vi "Live_Update_Bollean_indicator.vi"(8 "error in (no error)":errorcluster, 10 "Array 2":bool[](array[boolean]), 11 "Array":refnum<vi>[](array[refnum])) -> ()   [LabVIEW 2017]
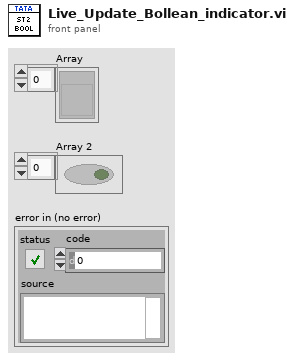
[diagram p1: front panel]
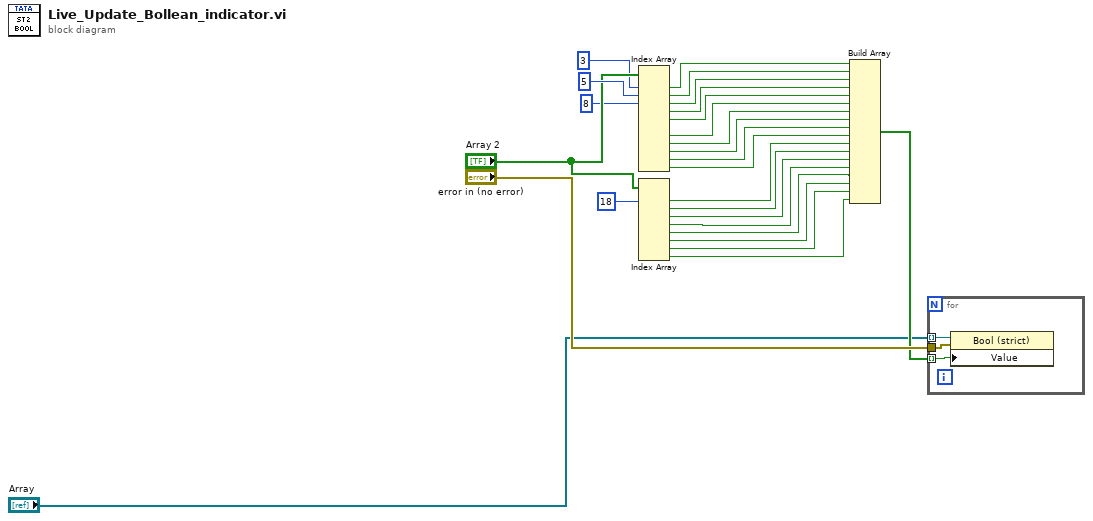
[diagram p0: block diagram]
diagram:
  n1 = Index Array(array="Array 2", index #1=3 ("index"), index #2=5 ("index"), index #3=8 ("index")) -> (element #1=w6:bool, element #2=w7:bool, element #3=w8:bool, element #4=w9:bool, element #5=w10:bool, element #7=w11:bool, element #8=w12:bool, element #9=w13:bool, element #10=w14:bool, element #11=w15:bool)  [unwired: 8 in, 1 out]
  n2 = Index Array(array="Array 2", index #1=18 ("index")) -> (element #1=w16:bool, element #2=w17:bool, element #3=w18:bool, element #4=w19:bool, element #5=w20:bool, element #6=w21:bool, element #7=w22:bool, element #8=w23:bool)  [unwired: 7 in]
  n3 = Build Array(w6, w7, w8, w9, w10, w11, w12, w13, w14, w15, w16, w17, w18, w19, w20, w21, w22, w23) -> (w25:bool[])
  n4 = for {
    tunnel: "Array" -> [w29] mode=indexing
    tunnel: w25 -> [w28] mode=indexing
    tunnel: "error in (no error)" -> [w27]
    n5 = property class="Bool (strict)"(reference=w29, error in=w27, "Value"=w28) -> ()  [unwired: 2 out]
  }
